vi "Configure Serial Bus (NRZ - Decode).vi"(0 "VISA resource name":refnum<visa-resource-name>, 1 "Word Size (8)":i32=8, 2 "Display Type (1: Word)":i32(ring)=1 items=["Bit", "Word"], 3 "Frame Size (8)":i32=8, 5 "Serial Bus Name (1: Serial Bus 1)":i32(ring)=1 items=["Serial Bus 1"=1, "Serial Bus 2"=2], 7 "Decode Base (0: Hexadecimal)":i32(ring) items=["Hexadecimal", "Unsigned Decimal", "ASCII", "Binary"], 9 "Bit Order (0: Most Significant Bit First)":i32(ring) items=["Most Significant Bit First", "Least Significant Bit First"], 11 "error in (no error)":errorcluster, 12 "Data Size (1)":i32=1, 13 "Header Size (0)":i32, 14 "Trailer Size (0)":i32) -> (4 "VISA resource name out":refnum<visa-resource-name>, 15 "error out":errorcluster)   [LabVIEW 2017, in "Agilent 2000 3000 X-Series.lvlib"]
doc: "Configures the decode setting of NRZ bus.\n\n<b>Note:</b>\nThis VI is only applicable for 3000T, 4000, 6000 X-Series."
uses:
  Agilent 2000 3000 X-Series.lvlib
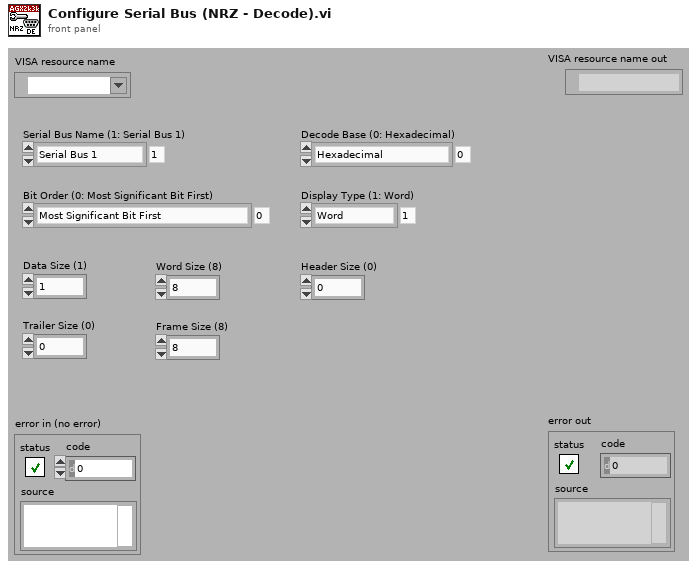
[diagram p1: front panel]
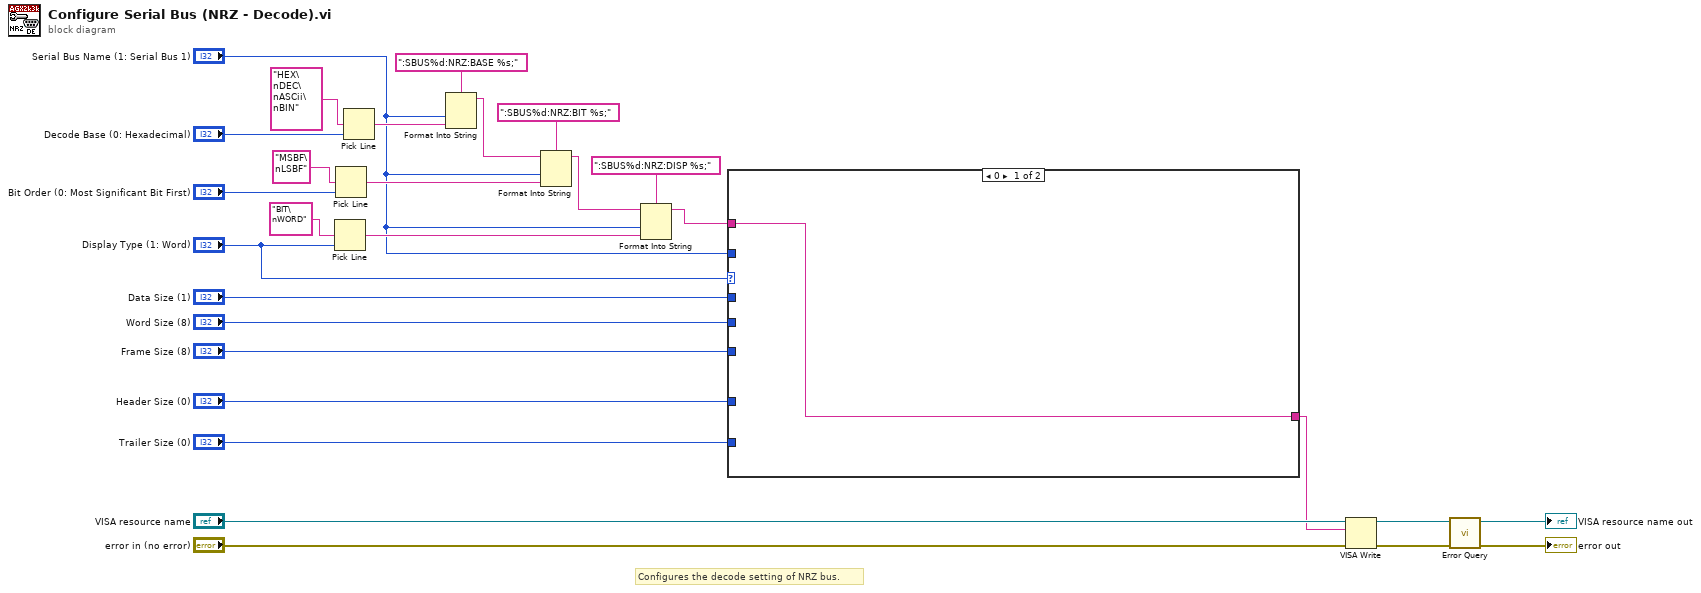
[diagram p0: block diagram]
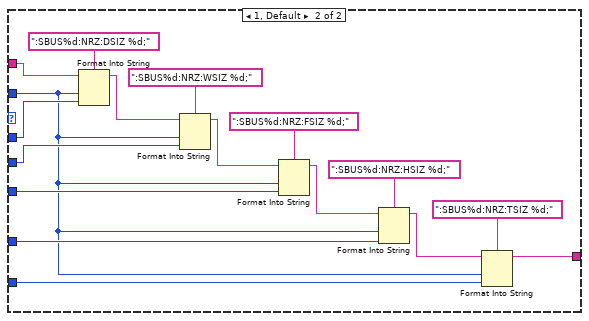
[diagram p2: hidden frame]
diagram:
  # "Configures the decode setting of NRZ bus."
  n1 = Pick Line(multi-line string="BIT\nWORD", line index="Display Type (1: Word)") -> (output string=w16:string)  [unwired: 1 in]
  n2 = Pick Line(multi-line string="MSBF\nLSBF", line index="Bit Order (0: Most Significant Bit First)") -> (output string=w25:string)  [unwired: 1 in]
  n3 = Pick Line(multi-line string="HEX\nDEC\nASCii\nBIN", line index="Decode Base (0: Hexadecimal)") -> (output string=w21:string)  [unwired: 1 in]
  n4 = Format Into String(format string=":SBUS%d:NRZ:BASE %s;", "Serial Bus Name (1: Serial Bus 1)", w21) -> (resulting string=w18:string)  [unwired: 2 in, 1 out]
  n5 = Format Into String(format string=":SBUS%d:NRZ:BIT %s;", initial string=w18, "Serial Bus Name (1: Serial Bus 1)", w25) -> (resulting string=w14:string)  [unwired: 1 in, 1 out]
  n6 = Format Into String(format string=":SBUS%d:NRZ:DISP %s;", initial string=w14, "Serial Bus Name (1: Serial Bus 1)", w16) -> (resulting string=w11:string)  [unwired: 1 in, 1 out]
  n7 = case shown="0" "Display Type (1: Word)" {
    tunnel: "Serial Bus Name (1: Serial Bus 1)" -> [_ w31]
    tunnel: w11 -> [w29 w45]
    tunnel: "Data Size (1)" -> [_ w44]
    tunnel: "Word Size (8)" -> [_ w41]
    tunnel: "Frame Size (8)" -> [_ w38]
    tunnel: "Header Size (0)" -> [_ w35]
    tunnel: "Trailer Size (0)" -> [_ w32]
    tunnel: [w29 w30] -> w1
    frame 0 {
    }
    frame 1, Default {
      n8 = Format Into String(format string=":SBUS%d:NRZ:DSIZ %d;", initial string=w45, w31, w44) -> (resulting string=w42:string)  [unwired: 1 in, 1 out]
      n9 = Format Into String(format string=":SBUS%d:NRZ:WSIZ %d;", initial string=w42, w31, w41) -> (resulting string=w40:string)  [unwired: 1 in, 1 out]
      n10 = Format Into String(format string=":SBUS%d:NRZ:FSIZ %d;", initial string=w40, w31, w38) -> (resulting string=w37:string)  [unwired: 1 in, 1 out]
      n11 = Format Into String(format string=":SBUS%d:NRZ:HSIZ %d;", initial string=w37, w31, w35) -> (resulting string=w34:string)  [unwired: 1 in, 1 out]
      n12 = Format Into String(format string=":SBUS%d:NRZ:TSIZ %d;", initial string=w34, w31, w32) -> (resulting string=w30:string)  [unwired: 1 in, 1 out]
    }
  }
  n13 = VISA Write(VISA resource name="VISA resource name", write buffer=w1, error in (no error)="error in (no error)") -> (VISA resource name out=w5:refnum<visa-resource-name>, error out=w4:errorcluster)  [unwired: 1 out]
  n14 = call "Error Query.vi"("error in (no error)"=w4, "VISA resource name"=w5) -> ("error out"=→"error out":errorcluster, "VISA resource name out"=→"VISA resource name out":refnum<visa-resource-name>)  [unwired: 6 in, 2 out]
